vi "Ex1_Graphs.vi"(6 "milliseconds to wait":u32(slide) scale=0.0..1000.0) -> (0 "Digital Waveform":dynamicdata(graph) caption="Analog Waveform 2", 3 "Analog Waveform":dynamicdata(graph) caption="Analog Waveform 1")   [LabVIEW 2020]
panel:
  out "Digital Waveform 4":dynamicdata(graph) caption="Analog Waveform 2"
  out "Analog Waveform 4":dynamicdata(graph) caption="Analog Waveform 1"
  out "Digital Waveform 3":dynamicdata(graph) caption="Analog Waveform 2"
  out "Analog Waveform 3":dynamicdata(graph) caption="Analog Waveform 1"
  out "Digital Waveform 2":dynamicdata(graph) caption="Analog Waveform 2"
  out "Analog Waveform 2":dynamicdata(graph) caption="Analog Waveform 1"
  in  "stop":bool
  # "Input Variables"
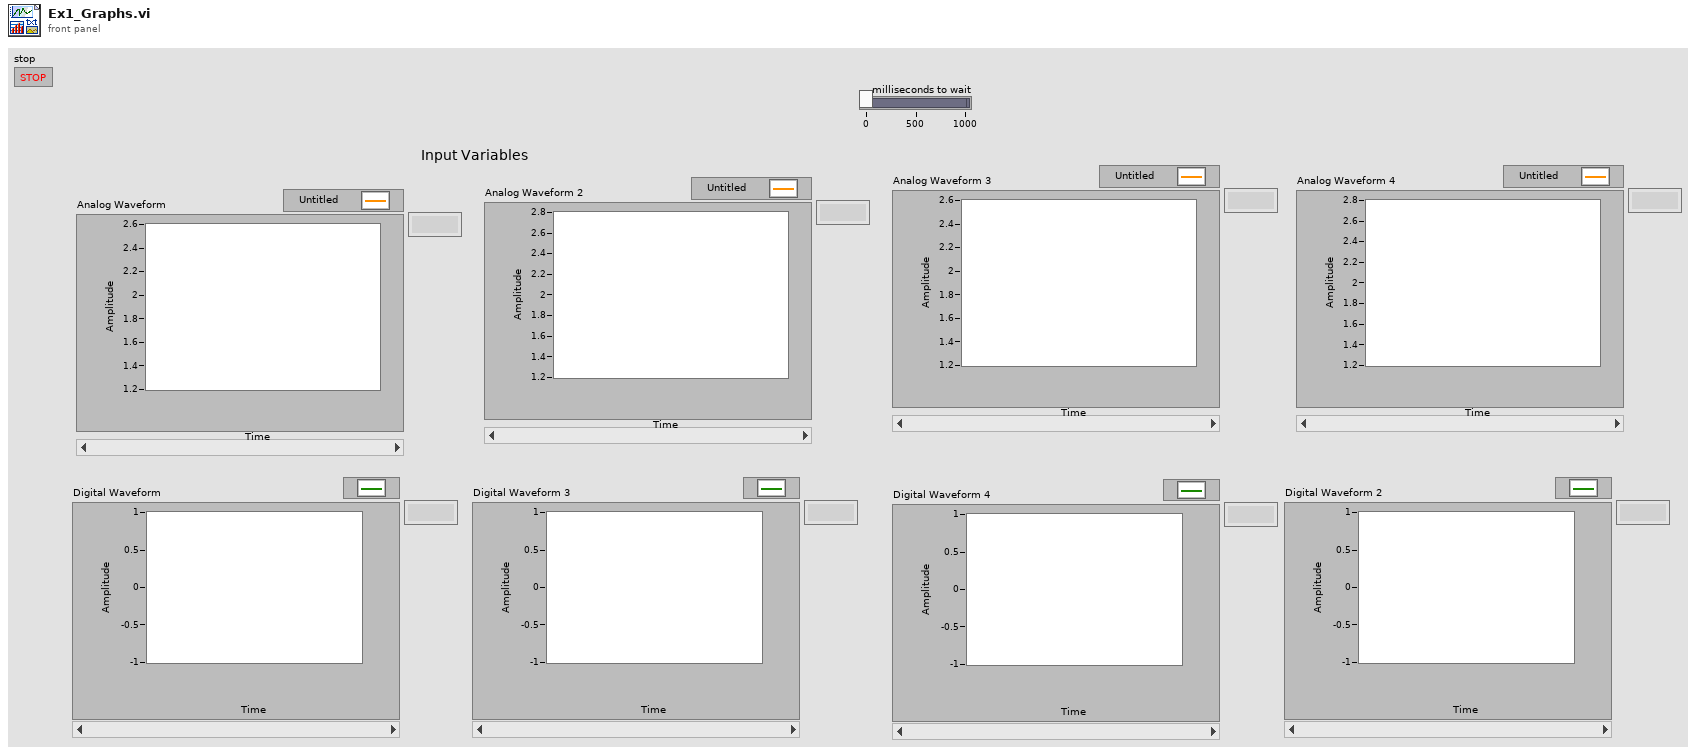
[diagram p1: front panel]
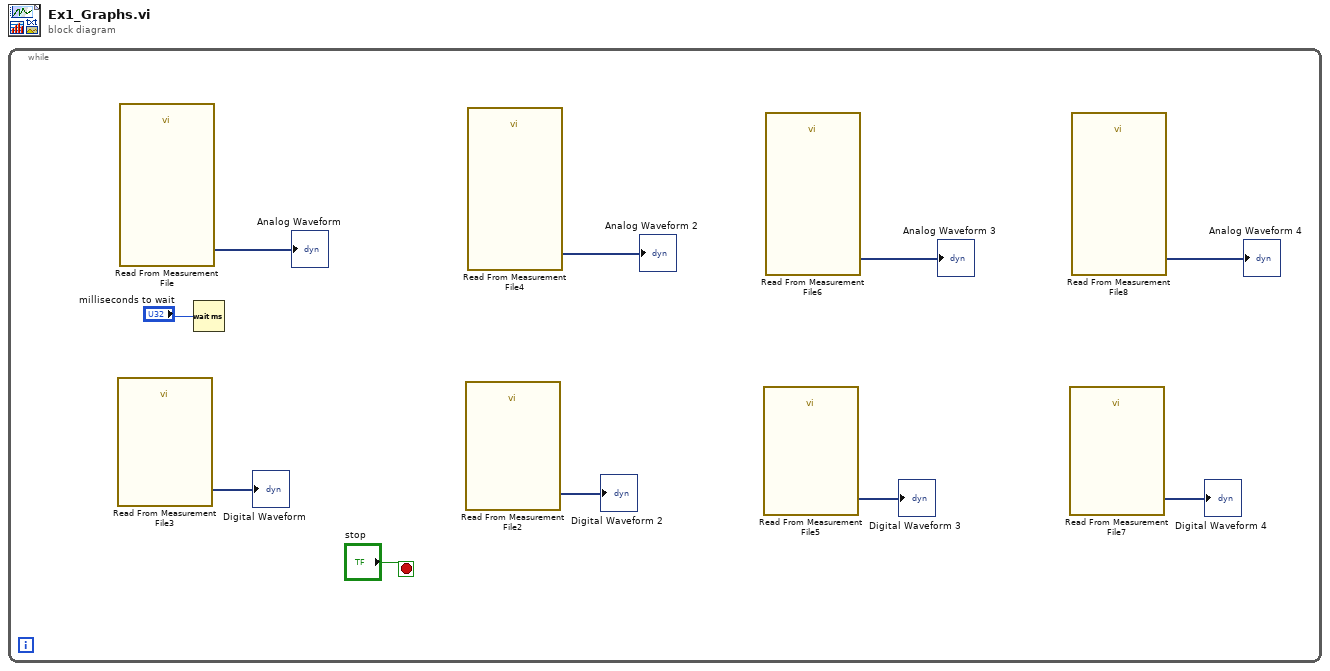
[diagram p0: block diagram]
diagram:
  n1 = while {
    stop <- "stop" stop-if-true
    n2 = call "Read From Measurement File3"() -> ("Signals"=→"Digital Waveform":dynamicdata)  [unwired: 6 in, 5 out]
    n3 = call "Read From Measurement File"() -> ("Signals"=→"Analog Waveform":dynamicdata)  [unwired: 6 in, 5 out]
    n4 = Wait (ms)(milliseconds to wait="milliseconds to wait") -> ()  [unwired: 1 out]
    n5 = call "Read From Measurement File2"() -> ("Signals"=→"Digital Waveform 2":dynamicdata)  [unwired: 6 in, 5 out]
    n6 = call "Read From Measurement File4"() -> ("Signals"=→"Analog Waveform 2":dynamicdata)  [unwired: 6 in, 5 out]
    n7 = call "Read From Measurement File5"() -> ("Signals"=→"Digital Waveform 3":dynamicdata)  [unwired: 6 in, 5 out]
    n8 = call "Read From Measurement File6"() -> ("Signals"=→"Analog Waveform 3":dynamicdata)  [unwired: 6 in, 5 out]
    n9 = call "Read From Measurement File7"() -> ("Signals"=→"Digital Waveform 4":dynamicdata)  [unwired: 6 in, 5 out]
    n10 = call "Read From Measurement File8"() -> ("Signals"=→"Analog Waveform 4":dynamicdata)  [unwired: 6 in, 5 out]
  }
